vi "旋转角通道.vi"() -> (0 "error out":errorcluster caption="错误输出", 1 "task out":refnum<k21> caption="任务输出")   [LabVIEW 2015]
uses:
  <vilib>/DAQmx/create/channels.llb/DAQmx Create Channel (CI-Count Edges).vi
  <resource>/objmgr/daqmx.rc
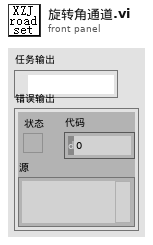
[diagram p1: front panel]
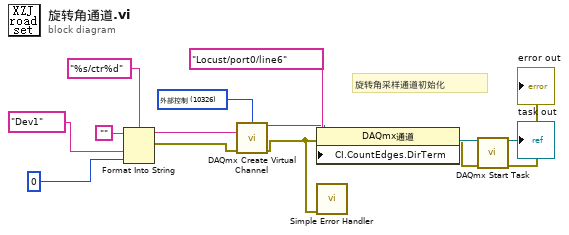
[diagram p0: block diagram]
diagram:
  w12 = 10326 items=["升值计数"=10128, "减值计数"=10124, "外部控制"=10326] ("count direction")
  # "旋转角采样通道初始化"
  n1 = Format Into String(format string="%s/ctr%d" ("格式字符串"), initial string="" ("初始字符串"), tag "Dev1" ("DAQmx设备名"), u32 0 ("数值")) -> (resulting string=w6:string, error out=w11:errorcluster)  [unwired: 1 in]
  n2 = call-poly <vilib>:"DAQmx Create Virtual Channel.vi"("count direction"=w12, "counter"=w6, "error in"=w11) -> ("task out"=w9:refnum<k21>, "error out"=w5:errorcluster)  [unwired: 11 in]
  n3 = property class="DAQmx通道"(reference=w9, error in=w5, "CI.CountEdges.DirTerm"=tag "Locust/port0/line6" ("CI.CountEdges.Term")) -> (reference out=w8:refnum<k21>, error out=w7:errorcluster)
  n4 = call <vilib>:"Simple Error Handler.vi"("error in (no error)"=w5) -> ()  [unwired: 4 in, 5 out]
  n5 = call <vilib>:"DAQmx Start Task.vi"("task/channels in"=w8, "error in"=w7) -> ("task out"=→"task out":refnum<k21>, "error out"=→"error out":errorcluster)  [unwired: 12 in]
